vi "Swerve Drive.vi"(0 "z":dbl(knob) scale=-1.0..1.0, 7 "y":dbl(slide) scale=-1.0..1.0, 11 "x":dbl(slide) scale=-1.0..1.0) -> ()   [LabVIEW 2016]
uses:
  <vilib>/Rock Robotics/WPI/ThirdParty/CanMotor/TalonSRX/WPI_CANTalonSRX_APIControlMode.ctl
  <vilib>/Rock Robotics/WPI/ThirdParty/CanMotor/TalonSRX/WPI_CANTalonSRX_APIFeedbackSelect.ctl
  Robot Global Data.vi
  <vilib>/Rock Robotics/Network Tables/NT Read Numeric Array.vi
  Apple Gyro/Apple Pi Gyro Library.lvlib
panel:
  in  "Recalc offsets":bool
  in  "milliseconds to wait":u32=5
  out "Loop Speed":u32
  in  "negate feedback sensor":bool
  in  "Recalc distance":bool=TRUE
  in  "Auto Controls":bool
  in  "Robot Centric":bool
  in  "Rot. Point X":dbl
  in  "Rot. Point Y":dbl
  in  "Deadband":dbl=0.04 format="%#_13g"
  in  "Debug?":bool
  in  "Motor":bool[](array[boolean])=[FALSE, FALSE, FALSE, FALSE]
  in  "PIDF":cluster{"P":dbl, "I":dbl, "D":dbl, "F":dbl}={"P"=2.0, "I"=0.0, "D"=0.0, "F"=0.0}
  in  "Robot Width":dbl=26.5
  in  "Robot Length":dbl=22.5
  in  "Reset Current":bool
  in  "Override NT?":bool
  in  "Gyro Select (Overide)":enum16{"IMU", "SPI", "Analog", "Navx"}(ring)=enum."Navx"
  # "SWERVE DRIVE\nVersion 4.0\nCory Lynch\nChris Garuti\nGavin Popkin\nApple Pi Robotics\nTeam 2067"
  # "FR"
  # "FL"
  # "BR"
  # "FL"
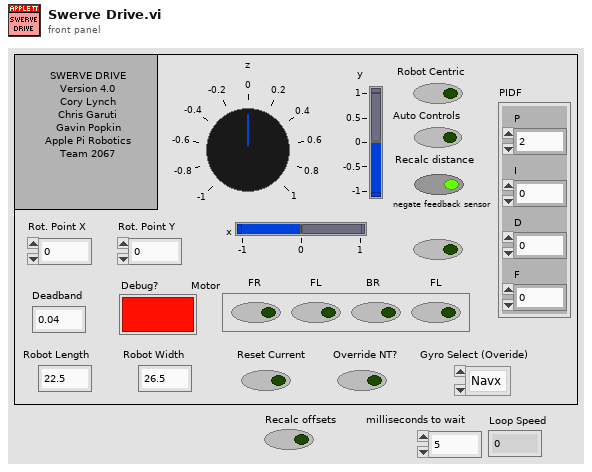
[diagram p1: front panel]
types:
  T1 = typedef "WPI_CANTalonSRX_APIFeedbackSelect.ctl" = enum16{"Digital Quadrature Encoder", "Analog Potentiometer", "Analog Encoder", "Count on Quad-A (Rising-Edge)", "Count on Quad-A (Falling-Edge)", "CTR Magnetic Enc (Absolute)", "CTR Magnetic Enc (Relative)", "Pulse Width"}
  T2 = typedef "WPI_CANTalonSRX_APIControlMode.ctl" = enum8{"Percent VBus", "Speed", "Position", "Slave", "Unchanged / Invalid", "Voltage Compensation", "Current", "Motion Profile", "Motion Magic"}
  T3 = typedef "WPI_MotorControlDeviceRef.ctl" = cluster{"DeviceStatus":errorcluster, "Type":T4, "PWM":cluster{"PWM Channel":T5, "DeadBand":T6}, "CAN":cluster{"Device Number":u8, "SetOutput VI Ref":variant, "GetOutput VI Ref":variant, "Enable VI Ref":variant, "Disable VI Ref":variant, "Data":variant}, "Invert":bool}
  T4 = typedef "WPI_MotorControlType.ctl" = enum16{"PWM", "CAN"}
  T5 = typedef "FPGA_DIOPWMChannel.ctl" = enum8{"PWM 0", "PWM 1", "PWM 2", "PWM 3", "PWM 4", "PWM 5", "PWM 6", "PWM 7", "PWM 8", "PWM 9", "PWM MXP 0", "PWM MXP 1", "PWM MXP 2", "PWM MXP 3", "PWM MXP 4", "PWM MXP 5", "PWM MXP 6", "PWM MXP 7", "PWM MXP 8", "PWM MXP 9", "Invalid"}
  T6 = typedef "WPI_PWMDeadband.ctl" = cluster{"Name":string, "maxPositivePwm":i32, "minPositivePwm":i32, "centerPwm":i32, "maxNegativePwm":i32, "minNegativePwm":i32, "angularRange":u16}
  T7 = typedef "WPI_CANTalonSRX_GlobalStatus.ctl" = cluster{"Applied Throttle":dbl, "Module Enabled":bool, "CAN Error":errorcluster, "Closed Loop Error":dbl, "Forward Limit Switch Closed":bool, "Reverse Limit Switch Closed":bool, "Sensor Position":dbl, "Sensor Velocity":dbl, "Current":dbl, "Sticky Fault - Over Temp":bool, "Sticky Fault - Under Voltage":bool, "Sticky Fault - Forward Limit":bool, "Sticky Fault - Reverse Limit":bool, "Sticky Fault - Forward Soft Limit":bool, "Sticky Fault - Reverse Soft Limit":bool, "Brake is Enabled":bool, "Encoder Position":dbl, "Encoder Velocity":dbl, "Encoder Index Count":dbl, "Encoder A Pin State":bool, "Encoder B Pin State":bool, "Encoder Index Pin State":bool, "Analog In":dbl, "Analog In Velocity":dbl, "Temperature (C)":dbl, "Battery Voltage":dbl, "Control 5 Is Supported":bool, "Current Profile Slot Select":dbl, "Pos Div 8":bool, "Vel Div 4":bool, "Pulse Width Position":i32, "Pulse Width Velocity":i32, "Pulse Width Rise To Rise (us)":i32, "Pulse Width Rise To Fall (us)":i32, "Mot Prof Active Is Under Run":bool, "Mot Prof Active Has Under Run":bool, "Mot Prof Active Is Last":bool, "Mot Prof Active Velocity Only":bool, "Mot Prof Active Is Valid":bool, "Mot Prof Buffer Is Full":bool, "Mot Prof Active Profile Slot Select":i32, "Mot Prof NextID":i32, "Mot Prof Count":i32, "Mot Prof Active Velocity":dbl, "Mot Prof Active Position":dbl, "Mot Prof Output Enable":i32, "UsageFrame":u32}
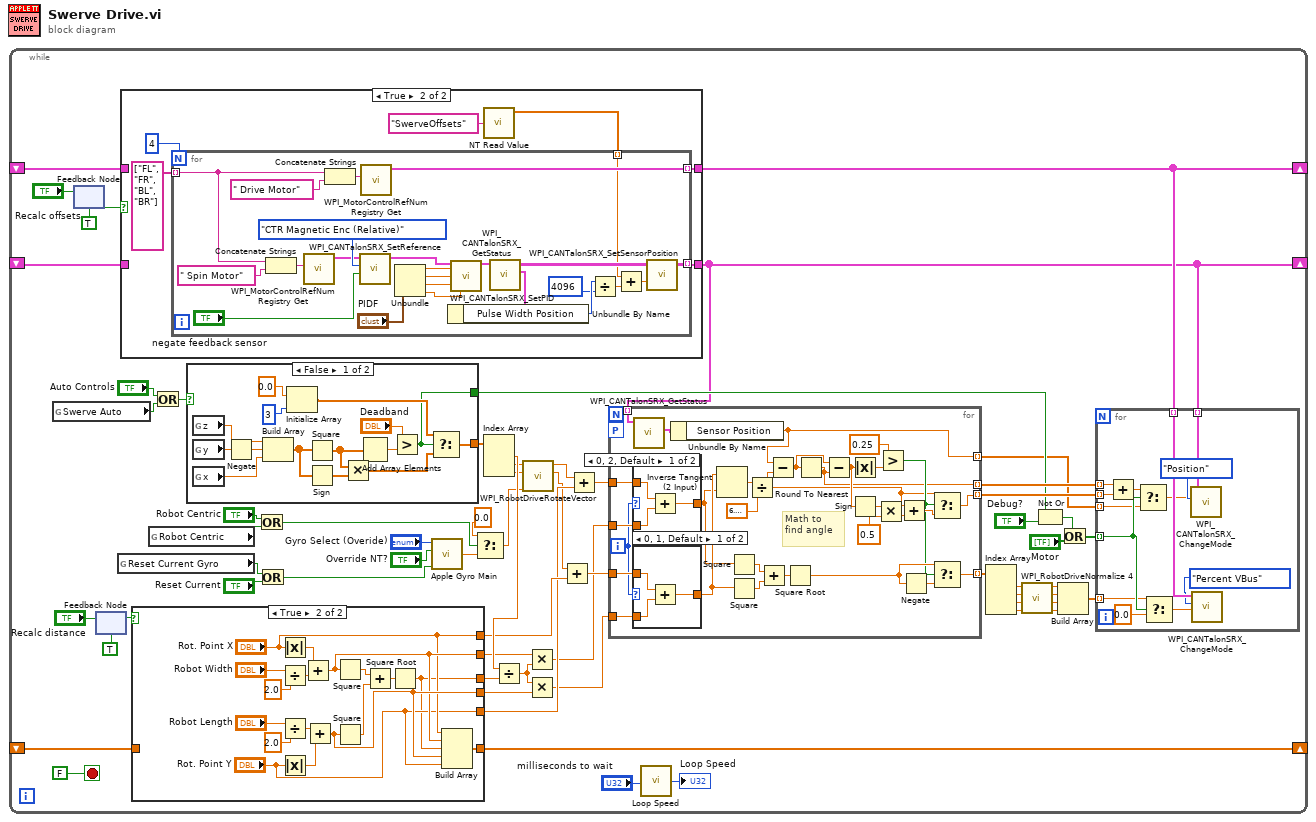
[diagram p0: block diagram]
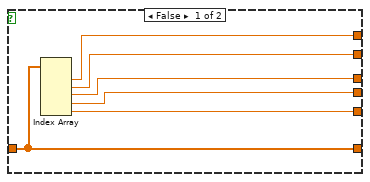
[diagram p3: hidden frame]
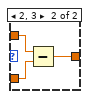
[diagram p4: hidden frame]
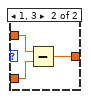
[diagram p5: hidden frame]
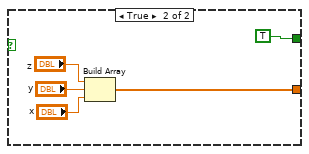
[diagram p6: hidden frame]
diagram:
  n1 = while {
    shift-right: [w52] -> _
    shift-left: _ -> [w51]
    shift-right: [w27] -> _
    shift-left: _ -> [w26]
    shift-right: [w24] -> _
    shift-left: _ -> [w25]
    stop <- FALSE stop-if-true
    n2 = global read "Robot Global Data.vi" "Swerve Auto"() -> (w11:bool)
    n3 = feedback-in #1("Recalc offsets") -> ()
    n4 = feedback #1(TRUE ("Do thung")) -> (w22:bool)
    n5 = feedback #2(TRUE ("Do thung")) -> (w15:bool)
    n6 = feedback-in #2("Recalc distance") -> ()
    n7 = global read "Robot Global Data.vi" "Reset Current Gyro"() -> (w13:bool)
    n8 = case shown="True" w22 {
      tunnel: [w64 w71] -> w24
      tunnel: [w65 w70] -> w27
      tunnel: w26 -> [w65 _]
      tunnel: w25 -> [w64 _]
      frame False {
      }
      frame True {
        n9 = call-poly <vilib>:"NT Read Value.vi"("Name"="SwerveOffsets") -> ("Numeric Array"=w66:dbl[])  [unwired: 9 in, 1 out]
        n10 = for {
          N: 4 -> [_]
          tunnel: string[] ["FL", "FR", "BL", "BR"] -> [w89] mode=indexing
          tunnel: [w86] -> w70 mode=indexing
          tunnel: [w78] -> w71 mode=indexing
          tunnel: w66 -> [w72] mode=indexing
          n11 = Concatenate Strings(w89, " Spin Motor" ("refnum name")) -> (w88:string)
          n12 = call <vilib>:"WPI_MotorControlRefNum Registry Get.vi"("refnum name"=w88) -> ("MotorControlDevRef"=w90:T3)  [unwired: 9 in, 1 out]
          n13 = Concatenate Strings(w89, " Drive Motor") -> (w87:string)
          n14 = call <vilib>:"WPI_CANTalonSRX_SetReference.vi"("Reverse Feedback Sensor"="negate feedback sensor", "Feedback Reference"=WPI_CANTalonSRX_APIFeedbackSelect."CTR Magnetic Enc (Relative)", "CAN Talon SRX Ref"=w90) -> ("CAN Talon SRX Ref"=w84:T3)  [unwired: 7 in, 1 out]
          n15 = call <vilib>:"WPI_MotorControlRefNum Registry Get.vi"("refnum name"=w87) -> ("MotorControlDevRef"=w86:T3)  [unwired: 9 in, 1 out]
          n16 = Unbundle("PIDF") -> ("P"=w91:dbl, "I"=w93:dbl, "D"=w92:dbl, "F"=w82:dbl)
          n17 = call <vilib>:"WPI_CANTalonSRX_SetPID.vi"("CAN Talon SRX Ref"=w84, "P"=w91, "I"=w93, "D"=w92, "F"=w82) -> ("CAN Talon SRX Ref"=w80:T3)  [unwired: 9 in, 1 out]
          n18 = call <vilib>:"WPI_CANTalonSRX_GetStatus.vi"("CAN Talon SRX Ref"=w80) -> ("Talon SRX Status"=w77:T7, "CAN Talon SRX Ref"=w79:T3)  [unwired: 8 in, 1 out]
          n19 = Unbundle By Name(w77) -> ("Pulse Width Position"=w75:i32)
          n20 = Divide(x=w75, y=4096) -> (x/y=w76:dbl)
          n21 = Add(x=w72, y=w76) -> (x+y=w73:dbl)
          n22 = call <vilib>:"WPI_CANTalonSRX_SetSensorPosition.vi"("New Sensor Position"=w73, "CAN Talon SRX Ref"=w79) -> ("CAN Talon SRX Ref"=w78:T3)  [unwired: 8 in, 1 out]
        }
      }
    }
    n23 = case shown="True" w15 {
      tunnel: [w113 w119] -> w58
      tunnel: [w110 "Rot. Point Y"] -> w54
      tunnel: [w114 "Rot. Point X"] -> w56
      tunnel: [w112 w115] -> w50
      tunnel: [w111 w120] -> w53
      tunnel: [w109 w116] -> w52
      tunnel: w51 -> [w109 _]
      frame False {
        n24 = Index Array(array=w109) -> (element #1=w114:dbl, element #2=w113:dbl, element #3=w112:dbl, element #4=w111:dbl, element #5=w110:dbl)  [unwired: 5 in]
      }
      frame True {
        n25 = Absolute Value(x="Rot. Point X") -> (abs(x)=w121:dbl)
        n26 = Divide(x="Robot Width", y=2.0) -> (x/y=w124:dbl)
        n27 = Divide(x="Robot Length", y=2.0) -> (x/y=w123:dbl)
        n28 = Absolute Value(x="Rot. Point Y") -> (abs(x)=w122:dbl)
        n29 = Add(x=w121, y=w124) -> (x+y=w119:dbl)
        n30 = Add(x=w123, y=w122) -> (x+y=w120:dbl)
        n31 = Square(x=w119) -> (x^2=w129:dbl)
        n32 = Square(x=w120) -> (x^2=w126:dbl)
        n33 = Add(x=w129, y=w126) -> (x+y=w130:dbl)
        n34 = Square Root(x=w130) -> (sqrt(x)=w115:dbl)
        n35 = Build Array("Rot. Point X", w119, w115, w120, "Rot. Point Y") -> (w116:dbl[])
      }
    }
    n36 = global read "Robot Global Data.vi" "Robot Centric"() -> (w19:bool)
    n37 = Or(x="Auto Controls", y=w11) -> (x .or. y?=w12:bool)
    n38 = case shown="False" w12 {
      tunnel: [w182 w193] -> w63
      tunnel: [w178 TRUE] -> w42
      frame False {
        n39 = global read "Robot Global Data.vi" "z"() -> (w176:dbl)
        n40 = global read "Robot Global Data.vi" "y"() -> (w177:dbl)
        n41 = global read "Robot Global Data.vi" "x"() -> (w174:dbl)
        n42 = Negate(x=w177) -> (-x=w175:dbl)
        n43 = Build Array(w176, w175, w174) -> (w186:dbl[])
        n44 = Initialize Array(0.0 ("element"), 3 ("dimension size")) -> (w188:dbl[])
        n45 = Square(x=w186) -> (x^2=w184:dbl[])
        n46 = Sign(1:w186) -> (0:w185:dbl[])
        n47 = Multiply(x=w184, y=w185) -> (x*y=w183:dbl[])
        n48 = Add Array Elements(numeric array=w184) -> (sum=w180:dbl)
        n49 = Greater?(x="Deadband", y=w180) -> (0:w178:bool)
        n50 = Select(t=w188, s=w178, f=w183) -> (s? t:f=w182:dbl[])
      }
      frame True {
        n51 = Build Array("z", "y", "x") -> (w193:dbl[])
      }
    }
    n52 = Or(x="Robot Centric", y=w19) -> (x .or. y?=w18:bool)
    n53 = Or(x=w13, y="Reset Current") -> (x .or. y?=w14:bool)
    n54 = call "Apple Gyro Main.vi"("Reset Current"=w14, "Override NT?"="Override NT?", "Gyro Select (Overide)"="Gyro Select (Overide)") -> ("Gyro Yaw Out"=w40:dbl)  [unwired: 1 in]
    n55 = Select(t=0.0, s=w18, f=w40) -> (s? t:f=w35:dbl)
    n56 = Index Array(array=w63) -> (element #1=w61:dbl, element #2=w34:dbl, element #3=w33:dbl)  [unwired: 3 in]
    n57 = Divide(x=w61, y=w50) -> (x/y=w60:dbl)
    n58 = call <vilib>:"WPI_RobotDriveRotateVector.vi"("Angle"=w35, "X"=w33, "Y"=w34) -> ("X'"=w29:dbl, "Y'"=w30:dbl)  [unwired: 7 out]
    n59 = Multiply(x=w58, y=w60) -> (x*y=w47:dbl)
    n60 = Multiply(x=w60, y=w53) -> (x*y=w46:dbl)
    n61 = Add(x=w29, y=w56) -> (x+y=w57:dbl)
    n62 = Add(x=w30, y=w54) -> (x+y=w55:dbl)
    n63 = for {
      tunnel: w55 -> [w161]
      tunnel: w47 -> [w160]
      tunnel: w57 -> [w159]
      tunnel: w46 -> [w158]
      tunnel: [w151] -> w10 mode=indexing
      tunnel: [w147] -> w45 mode=indexing
      tunnel: [w136] -> w44 mode=indexing
      tunnel: w24 -> [w137] mode=indexing
      tunnel: [w134] -> w28 mode=indexing
      workers-P: _ -> [_]
      i -> [w157]
      # "Math to\nfind angle"
      n64 = case shown="0, 2, Default" w157 {
        tunnel: w161 -> [w170 w173]
        tunnel: w160 -> [w169 w172]
        tunnel: [w168 w171] -> w132
        frame 0, 2, Default {
          n65 = Add(x=w170, y=w169) -> (x+y=w168:dbl)
        }
        frame 1, 3 {
          n66 = Subtract(x=w173, y=w172) -> (x-y=w171:dbl)
        }
      }
      n67 = case shown="0, 1, Default" w157 {
        tunnel: w159 -> [w164 w167]
        tunnel: w158 -> [w163 w166]
        tunnel: [w162 w165] -> w133
        frame 0, 1, Default {
          n68 = Add(x=w164, y=w163) -> (x+y=w162:dbl)
        }
        frame 2, 3 {
          n69 = Subtract(x=w167, y=w166) -> (x-y=w165:dbl)
        }
      }
      n70 = call <vilib>:"WPI_CANTalonSRX_GetStatus.vi"("CAN Talon SRX Ref"=w137) -> ("Talon SRX Status"=w138:T7)  [unwired: 8 in, 2 out]
      n71 = Unbundle By Name(w138) -> ("Sensor Position"=w134:dbl)
      n72 = Inverse Tangent (2 Input)(1:w132, 2:w133) -> (0:w149:dbl)
      n73 = Square(x=w132) -> (x^2=w155:dbl)
      n74 = Square(x=w133) -> (x^2=w156:dbl)
      n75 = Divide(x=w149, y=6.283185307179586) -> (x/y=w135:dbl)
      n76 = Add(x=w155, y=w156) -> (x+y=w154:dbl)
      n77 = Subtract(x=w134, y=w135) -> (x-y=w143:dbl)
      n78 = Square Root(x=w154) -> (sqrt(x)=w152:dbl)
      n79 = Round To Nearest(number=w143) -> (nearest integer value=w136:dbl)
      n80 = Subtract(x=w143, y=w136) -> (x-y=w144:dbl)
      n81 = Absolute Value(x=w144) -> (abs(x)=w140:dbl)
      n82 = Sign(1:w144) -> (0:w145:dbl)
      n83 = Multiply(x=w145, y=0.5) -> (x*y=w146:dbl)
      n84 = Greater?(x=0.25, y=w140) -> (0:w139:bool)
      n85 = Add(x=w135, y=w146) -> (x+y=w148:dbl)
      n86 = Negate(x=w152) -> (-x=w153:dbl)
      n87 = Select(t=w135, s=w139, f=w148) -> (s? t:f=w147:dbl)
      n88 = Select(t=w152, s=w139, f=w153) -> (s? t:f=w151:dbl)
    }
    n89 = call "Loop Speed.vi"("milliseconds to wait"="milliseconds to wait") -> ("Loop Speed"=→"Loop Speed":u32)
    n90 = Index Array(array=w10) -> (element #1=w9:dbl, element #2=w8:dbl, element #3=w7:dbl, element #4=w6:dbl)  [unwired: 4 in]
    n91 = call <vilib>:"WPI_RobotDriveNormalize 4.vi"("D"=w6, "C"=w7, "B"=w8, "A"=w9) -> ("D'"=w4:dbl, "C'"=w3:dbl, "B'"=w2:dbl, "A'"=w5:dbl)
    n92 = Not Or(1:"Debug?", 2:w42) -> (0:w41:bool)
    n93 = Build Array(w5, w2, w3, w4) -> (w1:dbl[])
    n94 = Or(x=w41, y="Motor") -> (x .or. y?=w49:bool[])
    n95 = for {
      tunnel: w45 -> [w105] mode=indexing
      tunnel: w24 -> [w108] mode=indexing
      tunnel: w27 -> [w107] mode=indexing
      tunnel: w49 -> [w100] mode=indexing
      tunnel: w44 -> [w104] mode=indexing
      tunnel: w28 -> [w99] mode=indexing
      tunnel: w1 -> [w96] mode=indexing
      n96 = Add(x=w104, y=w105) -> (x+y=w101:dbl)
      n97 = Select(t=w101, s=w100, f=w99) -> (s? t:f=w98:dbl)
      n98 = Select(t=w96, s=w100, f=0.0) -> (s? t:f=w106:dbl)
      n99 = call <vilib>:"WPI_CANTalonSRX_ChangeMode.vi"("Output"=w98, "Control Mode"=WPI_CANTalonSRX_APIControlMode."Position", "CAN Talon SRX Ref"=w108) -> ()  [unwired: 7 in, 2 out]
      n100 = call <vilib>:"WPI_CANTalonSRX_ChangeMode.vi"("Output"=w106, "Control Mode"=WPI_CANTalonSRX_APIControlMode."Percent VBus", "CAN Talon SRX Ref"=w107) -> ()  [unwired: 7 in, 2 out]
    }
  }
